vi "linear fit NaN.vi"(3 "Array 2":dbl[][](array[numeric]), 4 "Array":dbl[](array[numeric])) -> (1 "sloap":dbl, 2 "intercept":dbl)   [LabVIEW 2013, in "nan operations.lvlib"]
uses:
  nan operations.lvlib
  <vilib>/Analysis/6fits.llb/Curve Fitting Criteria.ctl
  <vilib>/Analysis/NI_AALPro.lvlib
panel:
  out "Waveform Graph":dbl[](graph)
  out "XY Graph":T1(graph)
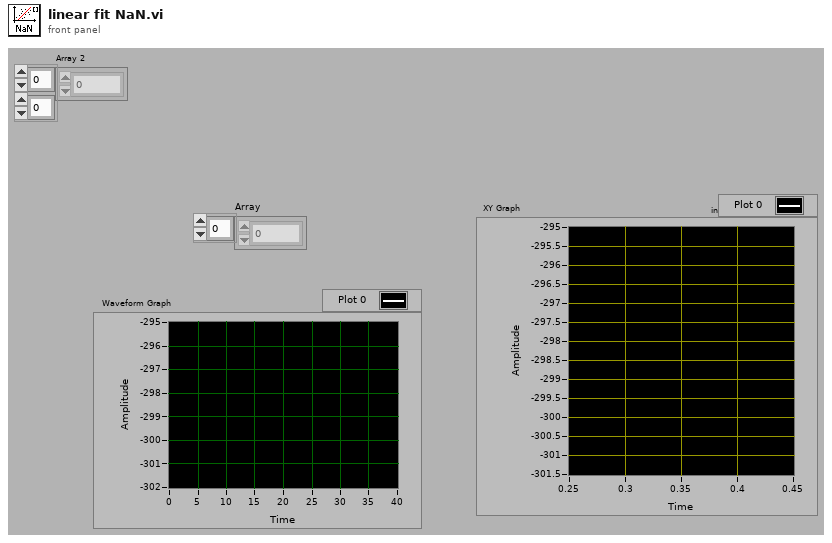
[diagram p1: front panel]
types:
  T1 = cluster{"Array 2":dbl[], "Best Linear Fit":dbl[]}[]
  T2 = typedef "NI_AALPro.lvlib/Curve Fitting Criteria.ctl" = u16
  T3 = cluster{"Array 2":dbl[], "Best Linear Fit":dbl[]}
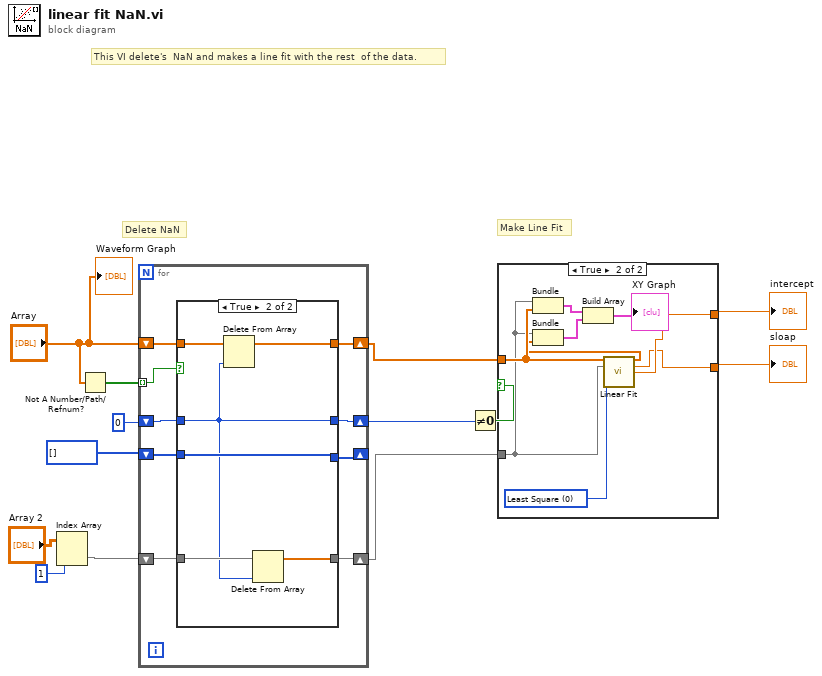
[diagram p0: block diagram]
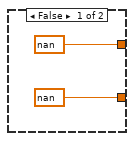
[diagram p2: hidden frame]
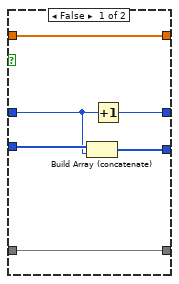
[diagram p3: hidden frame]
diagram:
  # "Make Line Fit"
  # "Delete NaN"
  # "This VI delete's  NaN and makes a line fit with the rest  of the data."
  n1 = Index Array(array="Array 2", index (col)=1 ("index (row)")) -> (element=w5:dbl[])  [unwired: 1 in]
  n2 = Not A Number/Path/Refnum?(number/path/refnum="Array") -> (NaN/Path/Refnum?=w13:bool[])
  n3 = for {
    tunnel: w13 -> [w21] mode=indexing
    shift-right: [w20] -> w2
    shift-left: "Array" -> [w22]
    shift-right: [w18] -> w9
    shift-left: 0 -> [w19]
    shift-right: [w16] -> _
    shift-left: i32[] [] -> [w17]
    shift-right: [w15] -> w4
    shift-left: w5 -> [w14]
    n4 = case shown="True" w21 {
      tunnel: w22 -> [w28 w34]
      tunnel: [w28 w33] -> w20
      tunnel: [w27 w29] -> w18
      tunnel: w19 -> [w24 w29]
      tunnel: w17 -> [w26 w32]
      tunnel: [w25 w32] -> w16
      tunnel: [w23 w30] -> w15
      tunnel: w14 -> [w23 w31]
      frame False {
        n5 = Build Array (concatenate)(w26, w24) -> (w25:i32[])
        n6 = Increment(x=w24) -> (x+1=w27:i32)
      }
      frame True {
        n7 = Delete From Array(array=w34, index=w29) -> (array with subset deleted=w33:dbl[])  [unwired: 1 in, 1 out]
        n8 = Delete From Array(array=w31, index=w29) -> (array with subset deleted=w30:dbl[])  [unwired: 1 in, 1 out]
      }
    }
  }
  n9 = Not Equal To 0?(x=w9) -> (x != 0?=w8:bool)
  n10 = case shown="True" w8 {
    tunnel: w2 -> [_ w42]
    tunnel: [nan ("intercept") w45] -> w11
    tunnel: [nan ("slope") w44] -> w10
    tunnel: w4 -> [_ w41]
    frame False {
    }
    frame True {
      w43 = T2 0 items=["Least Square", "Least Absolute Residual", "Bisquare"] ("method")
      n11 = Bundle("Array 2"=w41, "Array"=w42) -> (w39:cluster{"Array 2":dbl[], "Array":dbl[]})  [unwired: 1 in]
      n12 = call <vilib>:"Linear Fit.vi"("Y"=w42, "X"=w41, "method"=w43) -> ("Best Linear Fit"=w40:dbl[], "slope"=w44:dbl, "intercept"=w45:dbl)  [unwired: 8 in, 2 out]
      n13 = Bundle("Array 2"=w41, "Best Linear Fit"=w40) -> (w38:T3)  [unwired: 1 in]
      n14 = Build Array(w39, w38) -> (→"XY Graph":T1)
    }
  }
  "intercept" <- w11
  "sloap" <- w10
  "Waveform Graph" <- "Array"
